vi "Measurement UI.vi"() -> ()   [LabVIEW 2024, in "Analog Tachometer UI.lvlib"]
uses:
  Analog Tachometer UI.lvlib
panel:
  in  "channel":string="Dev1/ai0"
  out "tachometer waveforms":waveform(dbl)(graph)
  out "dt":dbl
  out "t0":dbl
  out "signal":dbl[](array[numeric])
  out "speed profile":cluster{"frequency":dbl[], "magnitude":dbl[]}(graph)
  in  "slope":u32(ring) items=["Rising", "Falling"]
  out "speed gage":dbl(knob) caption="RPM" scale=0.0..20000.0 scale format="%#_3p"
  in  "hysteresis":dbl=10.0 min=0.0 max=10.0 step=0.1 format="%#_g V"
  out "no tacho":bool
  in  "threshold":dbl=100.0 min=-100.0 max=100.0 step=0.1 format="%#_g V"
  in  "coupling":i32(ring)=10050 items=["AC"=10045, "DC"=10050, "GND"=10066]
  in  "IEPE current":dbl min=0.0 max=0.02 step=0.001 format="%#_g A"
  in  "max voltage":dbl=10.0 caption="maximum" min=-100.0 max=100.0 step=1.0 format="%#_g V"
  in  "channel I/O":tag="Dev1/ai0" caption="channel"
  in  "pulse/rev":i32=1 min=1 max=10000 step=1
  in  "sample rate":dbl=102400.0
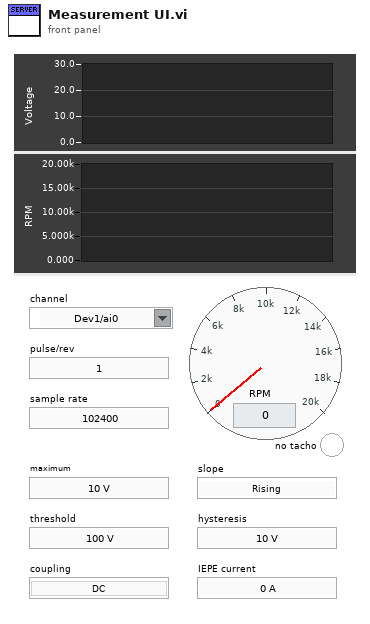
[diagram p1: front panel]
types:
  T1 = enum8{"Enabled", "Disabled", "Disabled and Grayed Out"}
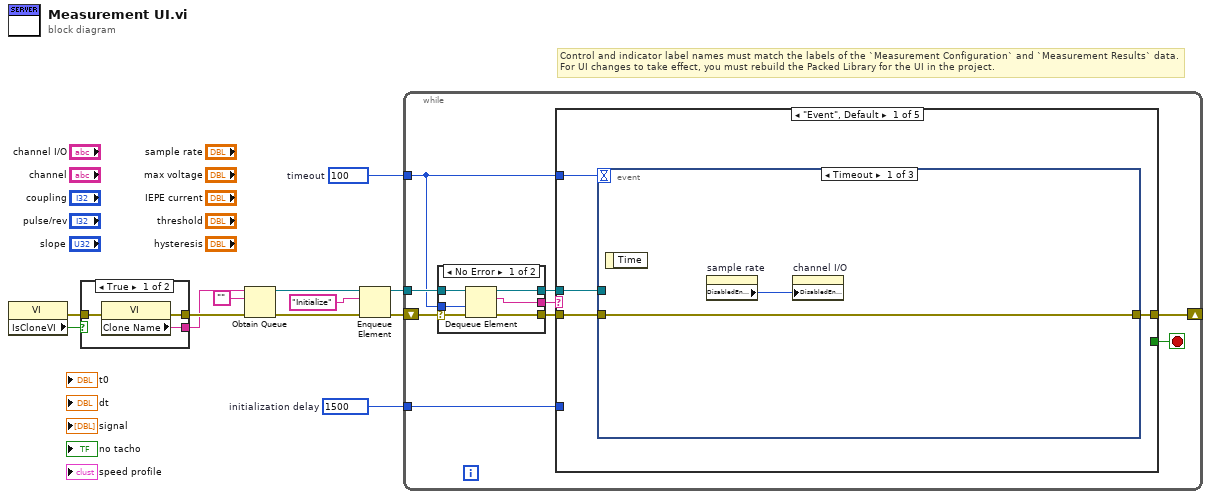
[diagram p0: block diagram]
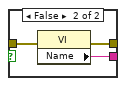
[diagram p2: hidden frame]
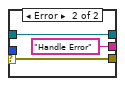
[diagram p3: hidden frame]
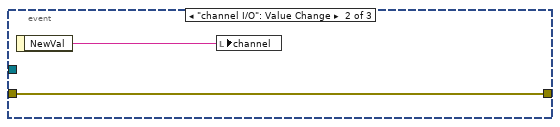
[diagram p4: hidden frame]
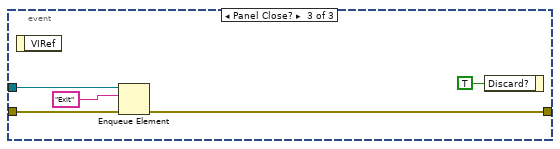
[diagram p5: hidden frame]
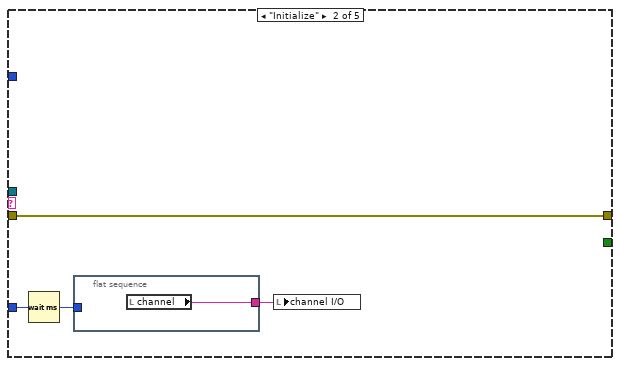
[diagram p6: hidden frame]
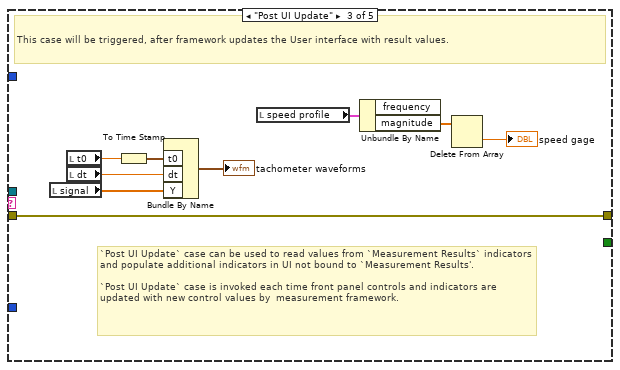
[diagram p7: hidden frame]
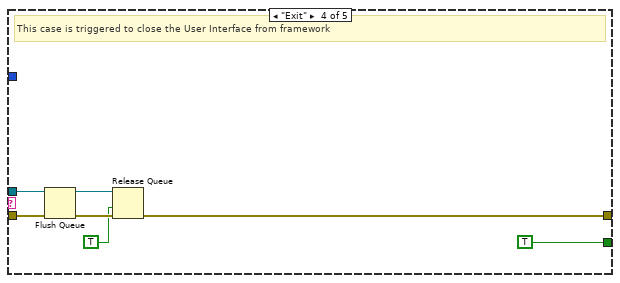
[diagram p8: hidden frame]
diagram:
  w1 = u32 1500  # initialization delay
  w2 = 100  # timeout
  # "Control and indicator label names must match the labels of the `Measurement Configuration` and `Measurement Results` data. \nFor UI changes to take effect, you must rebuild the Packed Library for the UI in the project."
  n1 = property class="VI"() -> (error out=w3:errorcluster, "IsCloneVI"=w4:bool)  [unwired: 2 in, 1 out]
  n2 = case shown="True" w4 {
    tunnel: [w15 w18] -> w12
    tunnel: [w14 w17] -> w11
    tunnel: w3 -> [w13 w16]
    frame True {
      n3 = property class="VI"(error in=w13) -> (error out=w15:errorcluster, "Clone Name"=w14:string)  [unwired: 1 in, 1 out]
    }
    frame False {
      n4 = property class="VI"(error in=w16) -> (error out=w18:errorcluster, "Name"=w17:string)  [unwired: 1 in, 1 out]
    }
  }
  n5 = Obtain Queue(name (unnamed)=w11, element data type="", error in (no error)=w12) -> (queue out=w8:refnum<queue>, error out=w10:errorcluster)  [unwired: 2 in, 1 out]
  n6 = Enqueue Element(queue=w8, element="Initialize", error in (no error)=w10) -> (queue out=w7:refnum<queue>, error out=w9:errorcluster)  [unwired: 1 in, 1 out]
  n7 = while {
    shift-right: [w22] -> _
    shift-left: w9 -> [w27]
    tunnel: w7 -> [w25]
    tunnel: w2 -> [w20]
    tunnel: w1 -> [w19]
    stop <- w21 stop-if-true
    n8 = case shown="No Error" w27 {
      selector: w27 -> [w33 w36]
      tunnel: [w32 w36] -> w26
      tunnel: w25 -> [w31 w35]
      tunnel: [w30 w35] -> w24
      tunnel: [w29 "Handle Error"] -> w23
      tunnel: w20 -> [w28 _]
      frame No Error {
        n9 = Dequeue Element(queue=w31, timeout in ms (-1)=w28, error in (no error)=w33) -> (queue out=w30:refnum<queue>, element=w29:string, error out=w32:errorcluster)  [unwired: 1 out]
      }
      frame Error {
      }
    }
    n10 = case shown="\"Event\", Default" w23 {
      tunnel: w26 -> [w39 w53 w63 w70 w71]
      tunnel: w24 -> [w38 _ _ w68 _]
      tunnel: [w40 w53 w63 w65 w71] -> w22
      tunnel: [_ _ _ TRUE _] -> w21
      tunnel: w20 -> [w37 _ _ _ _]
      tunnel: w19 -> [_ w52 _ _ _]
      frame "Event", Default {
        n11 = event shown="[0] Timeout" {
          selector: _ -> [_ _ _]
          dyn-events: _ -> [_ _ _]
          timeout: w37 -> [_ _ _]
          tunnel: [w42 w43 w47] -> w40
          tunnel: w39 -> [w42 w43 w48]
          tunnel: w38 -> [_ _ w46]
          event Timeout {
            n12 = event-data() -> ()  [unwired: 1 in, 1 out]
            n13 = property on="sample rate" class="DigNum (strict)"() -> ("DisabledEnum"=w41:T1)  [unwired: 2 in, 2 out]
            n14 = property on="channel I/O" class="DAQmxName"("DisabledEnum"=w41) -> ()  [unwired: 2 in, 2 out]
          }
          event "channel I/O": Value Change {
            n15 = event-data() -> ("NewVal"=w44:tag)  [unwired: 1 in]
            n16 = local write "channel"(w44) -> ()
          }
          event Panel Close? {
            n17 = event-data() -> ()  [unwired: 1 in, 1 out]
            n18 = Enqueue Element(queue=w46, element="Exit", error in (no error)=w48) -> (error out=w47:errorcluster)  [unwired: 1 in, 2 out]
            n19 = event-data("Discard?"=TRUE) -> ()  [unwired: 1 in, 1 out]
          }
        }
      }
      frame "Initialize" {
        n20 = Wait (ms)(milliseconds to wait=w52) -> (millisecond timer value=w51:u32)
        n21 = flat-sequence {
          tunnel: w51 -> [_]
          tunnel: [w54] -> w50
          frame #0 {
            n22 = local read "channel"() -> (w54:string)
          }
        }
        n23 = local write "channel I/O"(w50) -> ()
      }
      frame "Post UI Update" {
        # "`Post UI Update` case can be used to read values from `Measurement Results` indicators and populate additional indicators in UI not bound to `Measurement Results'.\n\n`Post UI Update` case is invoked each time front panel controls and indicators are updated with new control values by  measurement framework."
        # "This case will be triggered, after framework updates the User interface with result values."
        n24 = local read "signal"() -> (w59:dbl[])
        n25 = local read "t0"() -> (w61:dbl)
        n26 = local read "dt"() -> (w60:dbl)
        n27 = To Time Stamp(1:w61) -> (0:w62:timestamp)
        n28 = Bundle By Name("t0"=w62, "dt"=w60, "Y"=w59) -> (→"tachometer waveforms":waveform(dbl))  [unwired: 1 in]
        n29 = local read "speed profile"() -> (w58:cluster{"frequency":dbl[], "magnitude":dbl[]})
        n30 = Unbundle By Name(w58) -> ("magnitude"=w57:dbl[])  [unwired: 1 out]
        n31 = Delete From Array(array=w57) -> (deleted portion=→"speed gage":dbl)  [unwired: 2 in, 1 out]
      }
      frame "Exit" {
        # "This case is triggered to close the User Interface from framework"
        n32 = Flush Queue(queue=w68, error in (no error)=w70) -> (queue out=w67:refnum<queue>, error out=w66:errorcluster)  [unwired: 1 out]
        n33 = Release Queue(queue=w67, force destroy? (F)=TRUE, error in (no error)=w66) -> (error out=w65:errorcluster)  [unwired: 2 out]
      }
      frame "Handle Error" {
      }
    }
  }
